vi "count pulses.vi"(8 "error in":errorcluster, 11 "pulser":string(combo)) -> (0 "error out":errorcluster, 3 "pulser events":dbl format="%0.2f")   [LabVIEW 2016]
doc: "get number of pulser events sent to pxi chassis"
uses:
  <vilib>/DAQmx/read.llb/DAQmx Read (Counter DBL 1Chan 1Samp).vi
  <vilib>/DAQmx/miscellaneous.llb/DAQmx Fill In Error Info.vi
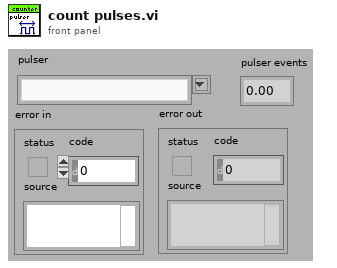
[diagram p1: front panel]
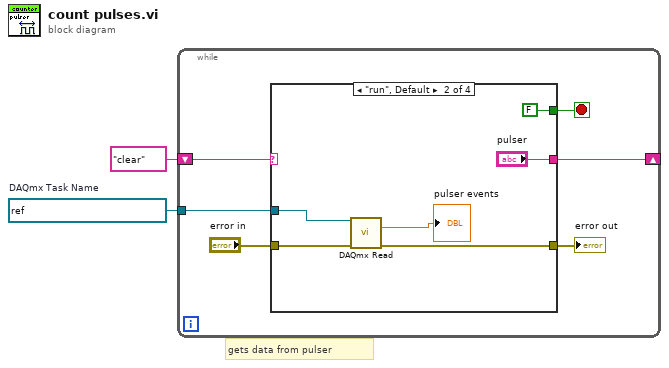
[diagram p0: block diagram]
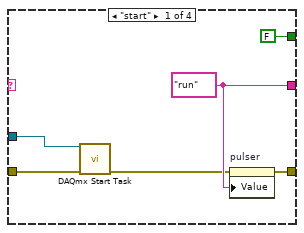
[diagram p2: hidden frame]
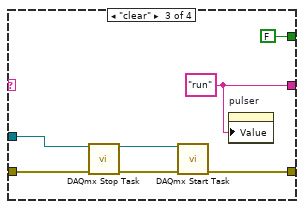
[diagram p3: hidden frame]
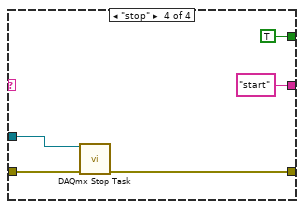
[diagram p4: hidden frame]
diagram:
  w2 = refnum<k21> "MyCountEdgesTask"  # DAQmx Task Name
  # "gets data from pulser"
  n1 = while {
    shift-right: [w5] -> _
    shift-left: "clear" ("pulser") -> [w8]
    tunnel: w2 -> [w6]
    stop <- w7 stop-if-true
    n2 = case shown="\"run\", Default" w8 {
      tunnel: [FALSE FALSE FALSE TRUE] -> w7
      tunnel: w6 -> [w13 w19 w25 w32]
      tunnel: [w12 "pulser" w23 "start" ("pulser")] -> w5
      tunnel: "error in" -> [w11 w16 w22 w29]
      tunnel: [w9 w15 w21 w28] -> w4
      frame "start" {
        w12 = "run" ("pulser")
        n3 = call <vilib>:"DAQmx Start Task.vi"("task/channels in"=w13, "error in"=w11) -> ("error out"=w10:errorcluster)  [unwired: 12 in, 1 out]
        n4 = property on="pulser" class="CmbBox"(error in=w10, "Value"=w12) -> (error out=w9:errorcluster)  [unwired: 1 in, 1 out]
      }
      frame "run", Default {
        n5 = call-poly <vilib>:"DAQmx Read.vi"("task/channels in"=w19, "error in"=w16) -> ("data"=→"pulser events":dbl, "error out"=w15:errorcluster)  [unwired: 11 in, 1 out]
      }
      frame "clear" {
        w23 = "run" ("pulser")
        n6 = call <vilib>:"DAQmx Stop Task.vi"("task/channels in"=w25, "error in"=w22) -> ("task out"=w26:refnum<k21>, "error out"=w27:errorcluster)  [unwired: 12 in]
        n7 = call <vilib>:"DAQmx Start Task.vi"("task/channels in"=w26, "error in"=w27) -> ("error out"=w21:errorcluster)  [unwired: 12 in, 1 out]
        n8 = property on="pulser" class="CmbBox"("Value"=w23) -> ()  [unwired: 2 in, 2 out]
      }
      frame "stop" {
        n9 = call <vilib>:"DAQmx Stop Task.vi"("task/channels in"=w32, "error in"=w29) -> ("error out"=w28:errorcluster)  [unwired: 12 in, 1 out]
      }
    }
    "error out" <- w4
  }
